vi "MonitorOperation.vi"(8 "Width":u32, 9 "Right":i16, 10 "Max - Min":dbl) -> (3 "Conversion":dbl)   [LabVIEW 2016]
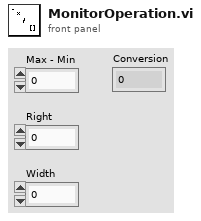
[diagram p1: front panel]
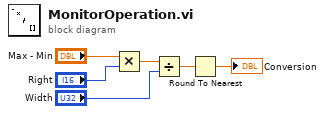
[diagram p0: block diagram]
diagram:
  n1 = Multiply(x="Max - Min", y="Right") -> (x*y=w4:dbl)
  n2 = Divide(x=w4, y="Width") -> (x/y=w3:dbl)
  n3 = Round To Nearest(number=w3) -> (nearest integer value=→"Conversion":dbl)
